vi "Close Hardware.vi"(8 "error in (no error)":errorcluster, 11 "Inst.AH2500 in":refnum<class "Inst.AH2500.lvclass">) -> (0 "error out":errorcluster, 3 "Inst.AH2500 out":refnum<class "Inst.AH2500.lvclass">)   [LabVIEW 2019, in "Inst.AH2500.lvclass"]
uses:
  Inst.AH2500.lvclass
  Inst.AH2500.lvclass/Inst.AH2500.ctl
  <userlib>/LevyLab/Instrument Framework/Instrument Types/VSource/Instrument.VSource.lvclass
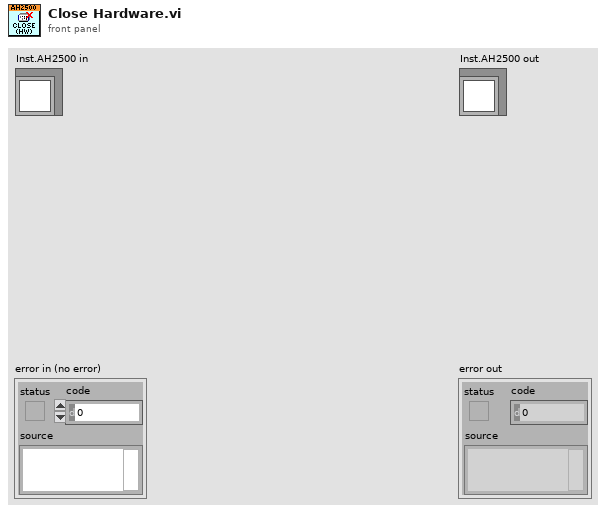
[diagram p1: front panel]
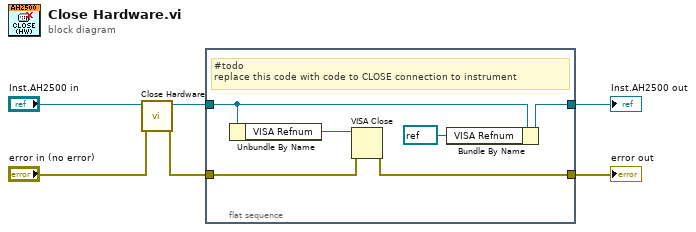
[diagram p0: block diagram]
diagram:
  n1 = call-parent "Close Hardware.vi"("error in (no error)"="error in (no error)", "Instrument in"="Inst.AH2500 in") -> ("error out"=w4:errorcluster, "Instrument out"=w2:refnum<class "Inst.AH2500.lvclass">)  [unwired: 8 in]
  n2 = flat-sequence {
    tunnel: w4 -> [w11]
    tunnel: [w10] -> w3
    tunnel: w2 -> [w8]
    tunnel: [w7] -> w1
    frame #0 {
      # "#todo\nreplace this code with code to CLOSE connection to instrument"
      n3 = Unbundle By Name(w8) -> ("VISA Refnum"=w12:refnum<visa-resource-name>)
      n4 = VISA Close(VISA resource name=w12, error in (no error)=w11) -> (error out=w10:errorcluster)
      n5 = Bundle By Name(cluster=w8, "VISA Refnum"=refnum<visa-resource-name> refnum) -> (w7:refnum<class "Inst.AH2500.lvclass">)
    }
  }
  "error out" <- w3
  "Inst.AH2500 out" <- w1
